vi "TCP_Server.vi"() -> ()   [LabVIEW 2019]
uses:
  9dddec59-2633-4920-86d0-fb84d7c00c5d.vi
panel:
  out "Array":string[](array[string])
  out "Boolean":bool
  out "Recepción":string
  in  "stop":bool
  in  "listening port":u16=4900
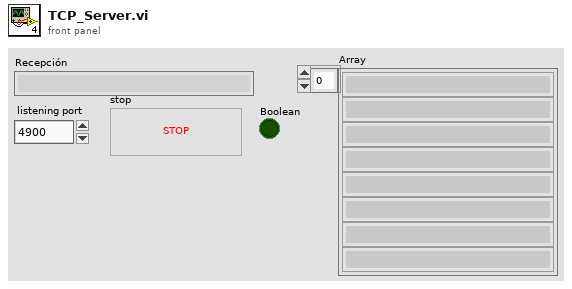
[diagram p1: front panel]
types:
  T1 = enum16{"Standard", "Buffered", "CRLF", "Immediate"}
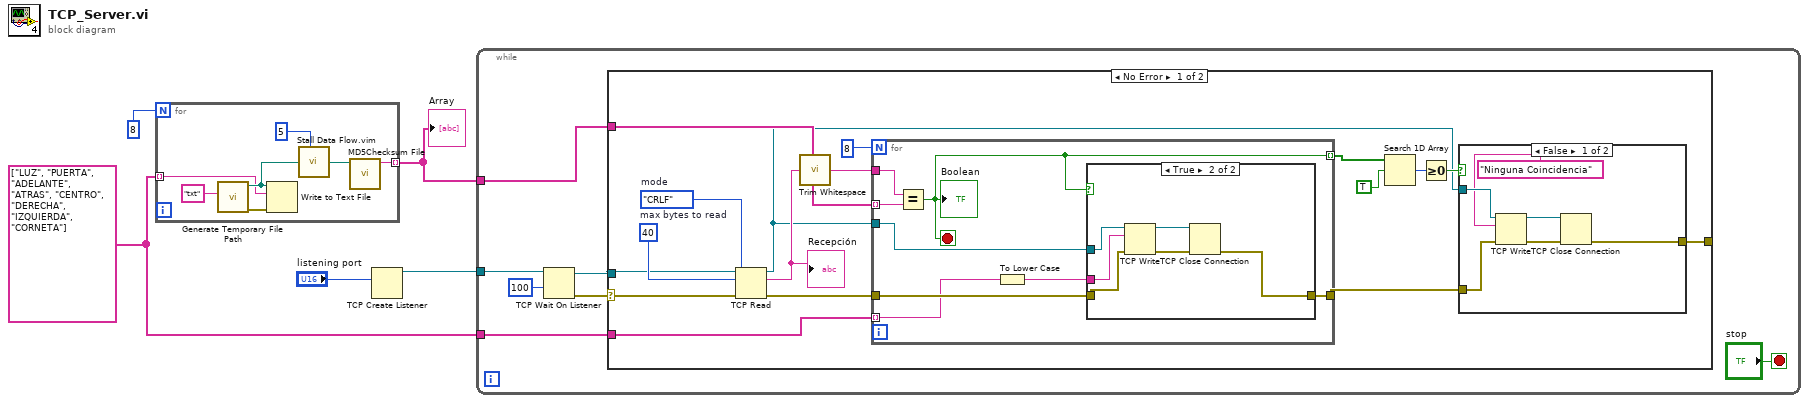
[diagram p0: block diagram]
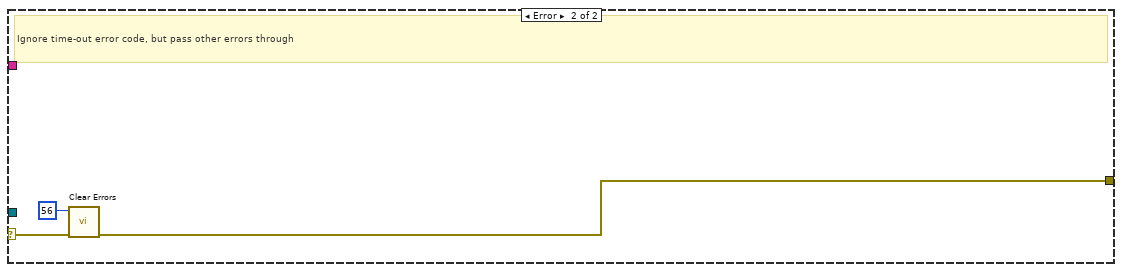
[diagram p4: hidden frame]
diagram:
  w1 = string[] ["LUZ", "PUERTA", "ADELANTE", "ATRAS", "CENTRO", "DERECHA", "IZQUIERDA", "CORNETA"]
  n1 = for {
    N: 8 -> [_]
    tunnel: w1 -> [w7] mode=indexing
    tunnel: [w6] -> w2 mode=indexing
    n2 = call <vilib>:"Generate Temporary File Path.vi"("Temporary File Extension (tmp)"="txt") -> ("error out"=w12:errorcluster, "Unique Temporary File Path"=w10:path)  [unwired: 9 in]
    n3 = Write to Text File(file (use dialog)=w10, text=w7, error in=w12) -> ()  [unwired: 1 in, 3 out]
    n4 = call "Stall Data Flow.vim"("value in"=w10, "milliseconds to wait"=u32 5) -> ("value out"=w11:path)  [unwired: 1 out]
    n5 = call <vilib>:"MD5Checksum File.vi"("Path"=w11) -> ("MD5 message-digest"=w6:string)  [unwired: 9 in, 1 out]
  }
  "Array" <- w2
  n6 = TCP Create Listener(10:"listening port") -> (3:w4:refnum<k5>)  [unwired: 4 in, 2 out]
  n7 = while {
    tunnel: w4 -> [w16]
    tunnel: w2 -> [w14]
    tunnel: w1 -> [w13]
    stop <- "stop" stop-if-true
    n8 = TCP Wait On Listener(9:100 ("timeout ms (25000)"), 11:w16) -> (0:w19:errorcluster, 4:w17:refnum<k5>)  [unwired: 2 in, 3 out]
    n9 = case shown="No Error" w19 {
      selector: w19 -> [w34 w61]
      tunnel: [w20 w60] -> _
      tunnel: w17 -> [w33 _]
      tunnel: w14 -> [w30 _]
      tunnel: w13 -> [w27 _]
      frame No Error {
        w36 = 40  # max bytes to read
        w35 = T1."CRLF"  # mode
        n10 = TCP Read(connection ID=w33, bytes to read=w36, error in (no error)=w34, 7:w35) -> (connection ID out=w22:refnum<k5>, data out=w29:string, error out=w28:errorcluster)  [unwired: 1 in]
        "Recepción" <- w29
        n11 = call <vilib>:"Trim Whitespace.vi"("string"=w29) -> ("trimmed string"=w32:string)  [unwired: 1 in]
        n12 = for {
          N: 8 -> [_]
          tunnel: w30 -> [w51] mode=indexing
          tunnel: w32 -> [w50]
          tunnel: w22 -> [w49]
          tunnel: w28 -> [w48]
          tunnel: [w45] -> w21
          tunnel: w27 -> [w47] mode=indexing
          tunnel: [w46] -> w24 mode=indexing
          stop <- w46 stop-if-true
          n13 = Equal?(x=w50, y=w51) -> (x = y?=w46:bool)
          "Boolean" <- w46
          n14 = To Lower Case(string=w47) -> (all lower case string=w44:string)
          n15 = case shown="True" w46 {
            tunnel: w49 -> [_ w56]
            tunnel: w48 -> [w52 w55]
            tunnel: [w52 w54] -> w45
            tunnel: w44 -> [_ w53]
            frame False {
            }
            frame True {
              n16 = TCP Write(connection ID=w56, data in=w53, error in (no error)=w55) -> (connection ID out=w58:refnum<k5>, error out=w57:errorcluster)  [unwired: 1 in, 1 out]
              n17 = TCP Close Connection(connection ID=w58, error in (no error)=w57) -> (error out=w54:errorcluster)  [unwired: 1 in, 1 out]
            }
          }
        }
        n18 = Search 1D Array(1D array=w24, element=TRUE) -> (index of element=w25:i32)  [unwired: 1 in]
        n19 = Greater Or Equal To 0?(x=w25) -> (x >= 0?=w23:bool)
        n20 = case shown="False" w23 {
          tunnel: w22 -> [w40 _]
          tunnel: w21 -> [w39 w43]
          tunnel: [w37 w43] -> w20
          frame False {
            n21 = TCP Write(connection ID=w40, data in="Ninguna Coincidencia", error in (no error)=w39) -> (connection ID out=w42:refnum<k5>, error out=w41:errorcluster)  [unwired: 1 in, 1 out]
            n22 = TCP Close Connection(connection ID=w42, error in (no error)=w41) -> (error out=w37:errorcluster)  [unwired: 1 in, 1 out]
          }
          frame True {
          }
        }
      }
      frame Error {
        # "Ignore time-out error code, but pass other errors through"
        n23 = call <vilib>:"Clear Errors.vi"("error in (no error)"=w61, "specific error code to clear (0: all)"=56) -> ("error out"=w60:errorcluster)  [unwired: 4 in, 1 out]
      }
    }
  }
